vi "resultsColumnsMultirun.vi"(10 "chValuesIn":string[](array[string]), 11 "chNamesIn":string[](array[string])) -> (2 "chValuesOut":string[](array[string]), 3 "chNamesOut":string[](array[string]))   [LabVIEW 2020]
uses:
  Globals/Meas_global.vi
  Globals/Trav_pos_global.vi
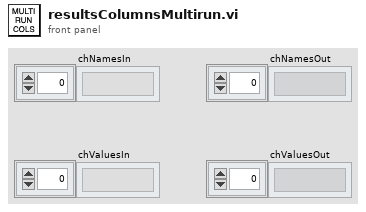
[diagram p1: front panel]
types:
  T1 = typedef "Post_Process.ctl" = enum16{"Take New Data", "Post Process Raw Data File"}
  T2 = enum32{"Bad", "Idle", "Run top level", "Running"}
  T3 = typedef "Traverse_cluster.ctl" = cluster{"Start X":sgl, "Start Y":sgl, "Start Z":sgl, "End X":sgl, "End Y":sgl, "End Z":sgl, "nPoints":i32, "Spacing":T4, "Filename":path, "Tunnel Speed":dbl, "Averaging time (mins)":dbl, "Extra Commands":string, "Carrier_1 Q (l/min)":dbl, "Carrier_2 Q (l/min)":dbl, "Trace Gas Concentration (%)":dbl, "Specific Arguments":string, "Comments":string, "Row No":i32, "Row Type Selector":T5, "EstCompl":string, "Row Duration (mins)":dbl, "nValidPoints":i32, "Meas Setup File":string}
  T4 = typedef "Spacing.ctl" = enum16{"Linear", "Log", "Gauss", "Specified", "N/A"}
  T5 = typedef "Multi_run_mode.ctl" = enum16{"Move Traverse Only", "Set Tunnel Speed Only", "Set Source Only", "Set Measurement Conditions", "Single Measurement", "Vertical Profile", "Lateral Profile", "Longitudinal Profile", "Multi-Axis Profile", "Explore Volume", "Auto Calibrate", "Meas Fast FID Bkgnd", "Check Beam Power", "Scanning Valve Measurement", "Run VI Named:", "Set ADAM Ch", "Wait (minutes)", "Send Message", "Synchronize With:", "Fall Back to this Row", "Turn Off Row Repeating", "Traverse 3D Volume", "Blank Row", "Jump to Fall Back Row"}
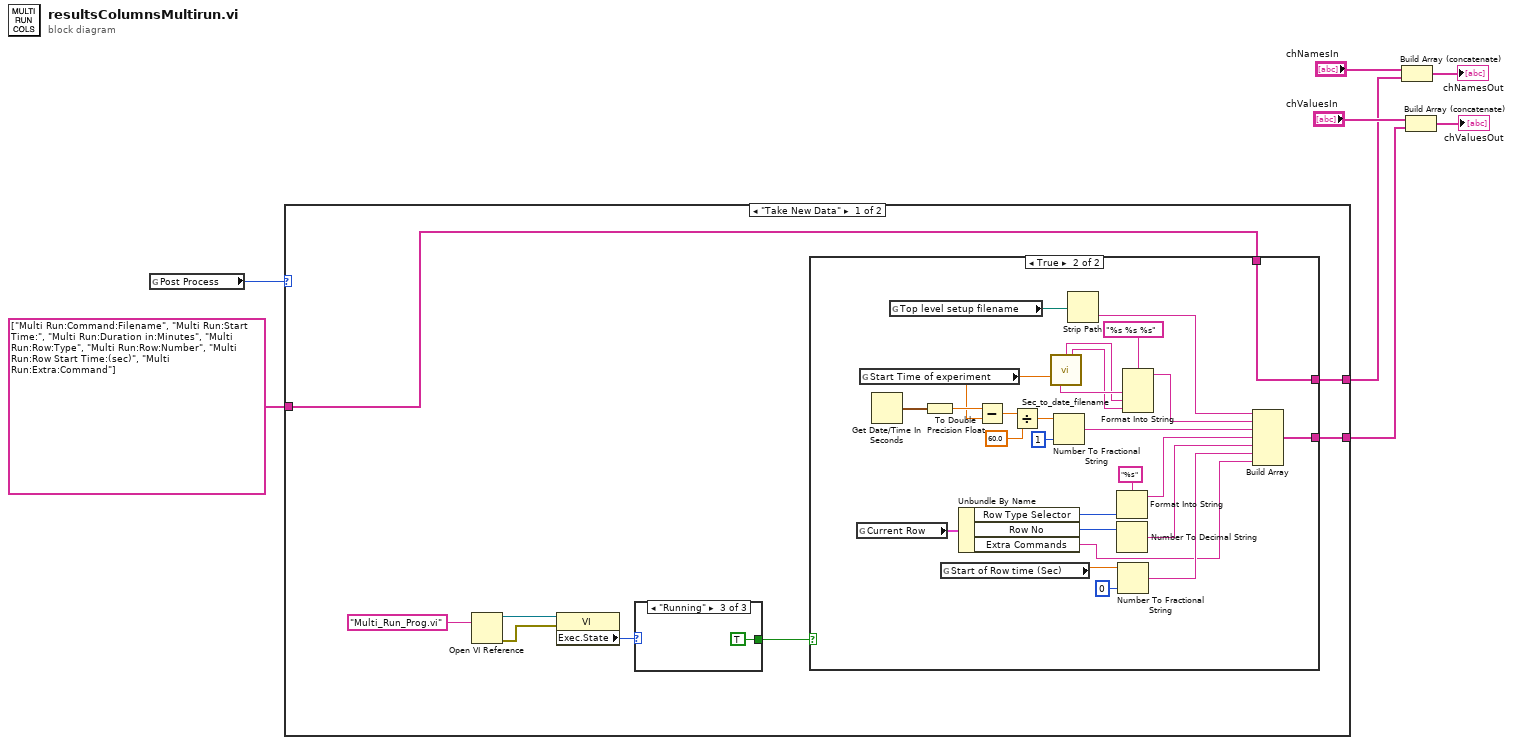
[diagram p0: block diagram]
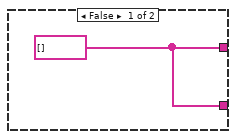
[diagram p2: hidden frame]
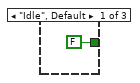
[diagram p3: hidden frame]
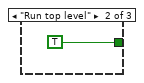
[diagram p4: hidden frame]
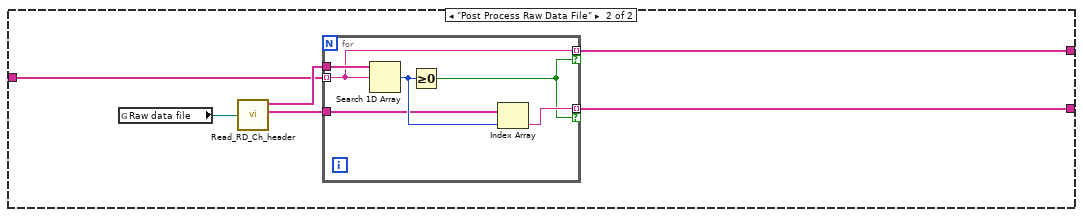
[diagram p5: hidden frame]
diagram:
  n1 = global read "Meas_global.vi" "Post Process"() -> (w3:T1)
  n2 = case shown="\"Take New Data\"" w3 {
    tunnel: [w16 w50] -> w2
    tunnel: string[] ["Multi Run:Command:Filename", "Multi Run:Start Time:", "Multi Run:Duration in:Minutes", "Multi Run:Row:Type", "Multi Run:Row:Number", "Multi Run:Row Start Time:(sec)", "Multi Run:Extra:Command"] ("appended array") -> [w10 w51]
    tunnel: [w9 w49] -> w1
    frame "Take New Data" {
      n3 = Open VI Reference(vi path="Multi_Run_Prog.vi") -> (vi reference=w13:refnum<vi>, error out=w14:errorcluster)  [unwired: 5 in]
      n4 = property class="VI"(reference=w13, error in=w14) -> ("Exec.State"=w15:T2)  [unwired: 2 out]
      n5 = case shown="\"Running\"" w15 {
        tunnel: [FALSE TRUE TRUE] -> w11
        frame "Idle", Default {
        }
        frame "Run top level" {
        }
        frame "Running" {
        }
      }
      n6 = case shown="True" w11 {
        tunnel: [w17 w36] -> w16
        tunnel: w10 -> [_ w21]
        tunnel: [w17 w21] -> w9
        frame False {
          w17 = string[] [] ("appended array")
        }
        frame True {
          n7 = global read "Trav_pos_global.vi" "Current Row"() -> (w42:T3)
          n8 = global read "Meas_global.vi" "Start Time of experiment"() -> (w32:dbl)
          n9 = Get Date/Time In Seconds() -> (seconds since 1Jan1904=w22:timestamp)
          n10 = global read "Trav_pos_global.vi" "Top level setup filename"() -> (w35:path)
          n11 = To Double Precision Float(number=w22) -> (double precision float=w33:dbl)
          n12 = global read "Trav_pos_global.vi" "Start of Row time (Sec)"() -> (w26:dbl)
          n13 = Unbundle By Name(w42) -> ("Row Type Selector"=w41:T5, "Row No"=w38:i32, "Extra Commands"=w23:string)
          n14 = Subtract(x=w33, y=w32) -> (x-y=w31:dbl)
          n15 = Divide(x=w31, y=60.0) -> (x/y=w29:dbl)
          n16 = call "Sec_to_date_filename.vi"("ss1904"=w32) -> ("shortDayName"=w19:string, "HH:MM"=w18:string, "YYYY-mm-DD"=w20:string)  [unwired: 5 in, 7 out]
          n17 = Number To Fractional String(number=w29, precision (6)=i16 1) -> (F-format string=w27:string)  [unwired: 2 in]
          n18 = Strip Path(path=w35) -> (name=w34:string)  [unwired: 1 out]
          n19 = Format Into String(format string="%s", w41) -> (resulting string=w39:string)  [unwired: 2 in, 1 out]
          n20 = Number To Decimal String(number=w38) -> (decimal integer string=w37:string)  [unwired: 1 in]
          n21 = Number To Fractional String(number=w26, precision (6)=i16 0) -> (F-format string=w24:string)  [unwired: 2 in]
          n22 = Format Into String(format string="%s %s %s", w20, w19, w18) -> (resulting string=w43:string)  [unwired: 2 in, 1 out]
          n23 = Build Array(w34, w43, w27, w39, w37, w24, w23) -> (w36:string[])
        }
      }
    }
    frame "Post Process Raw Data File" {
      n24 = global read "Meas_global.vi" "Raw data file"() -> (w48:path)
      n25 = call "Read_RD_Ch_header.vi"("Raw data file"=w48) -> ("Ch Name Out"=w53:string[], "Ch Values"=w52:string[])  [unwired: 2 out]
      n26 = for {
        tunnel: w53 -> [w59]
        tunnel: w52 -> [w57]
        tunnel: [w56] -> w50 mode=indexing if=w54
        tunnel: w51 -> [w55] mode=indexing
        tunnel: [w55] -> w49 mode=indexing if=w54
        n27 = Search 1D Array(1D array=w59, element=w55) -> (index of element=w58:i32)  [unwired: 1 out]
        n28 = Greater Or Equal To 0?(x=w58) -> (x >= 0?=w54:bool)
        n29 = Index Array(array=w57, index=w58) -> (element=w56:string)
      }
    }
  }
  n30 = Build Array (concatenate)("chNamesIn", w1) -> (→"chNamesOut":string[])
  n31 = Build Array (concatenate)("chValuesIn", w2) -> (→"chValuesOut":string[])
